vi "refresh table model.vi"(7 "engine configuration":refnum<class "engine configuration.lvclass">, 8 "error in":errorcluster, 9 "avail tags":refnum<vi>, 10 "chan table":refnum<vi>, 11 "TDMS datalogger configuration":refnum<class "TDMS datalogger configuration.lvclass">) -> (0 "error out":errorcluster, 3 "TDMS datalogger configuration out":refnum<class "TDMS datalogger configuration.lvclass">, 5 "engine configuration out":refnum<class "engine configuration.lvclass">)   [LabVIEW 2013, in "TDMS datalogger editor node.lvclass"]
uses:
  TDMS datalogger editor node.lvclass
  <vilib>/NI/TBM Modules/TDMS Datalogger/module/configuration/TDMS datalogger configuration.lvclass
  <vilib>/NI/Module Execution Interface/Engine Configuration/engine configuration.lvclass
  <vilib>/NI/Tag Bus Module Framework/root configuration/TBM configuration.lvclass/TBM configuration.ctl
  <vilib>/NI/TBM Modules/TDMS Datalogger/module/configuration/TDMS datalogger configuration.lvclass/TDMS datalogger configuration.ctl
  <vilib>/NI/Tag Bus/tag/tag descriptor.lvclass/tag descriptor.ctl
  <vilib>/NI/Module Execution Interface/Engine Configuration/engine configuration.lvclass/engine configuration.ctl
  <vilib>/NI/Tag Bus/tag/read tag name.vi
  <vilib>/NI/Tag Bus/tag/read data type.vi
  <vilib>/NI/Tag Bus Module Framework/root configuration/Read instance name.vi
  <vilib>/NI/TBM Modules/TDMS Datalogger/module/configuration/Read channels.vi
  <vilib>/NI/Tag Bus Module Framework/root configuration/create GUID.vi
  <vilib>/NI/Tag Bus Module Framework/channel/TBM channel.lvclass
  <vilib>/NI/Tag Bus/tag/tag descriptor.lvclass
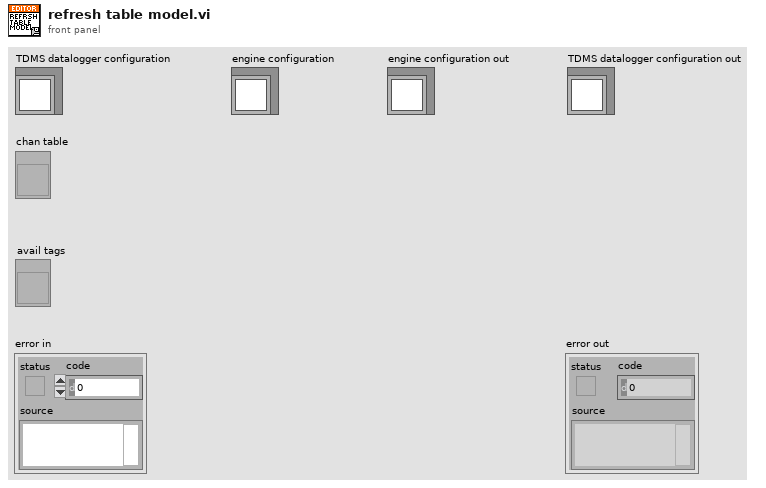
[diagram p1: front panel]
types:
  T1 = typedef "tag bus.lvlib/tag descriptor.lvclass/Data Type.ctl" = enum16{"Double", "Single", "I64", "I32", "I16", "I8", "U64", "U32", "U16", "U8", "Boolean", "String", "Array of Double", "Array of Single", "Array of I64", "Array of I32", "Array of I16", "Array of I8", "Array of U64", "Array of U32", "Array of U16", "Array of U8", "Array of Boolean", "Array of String"}
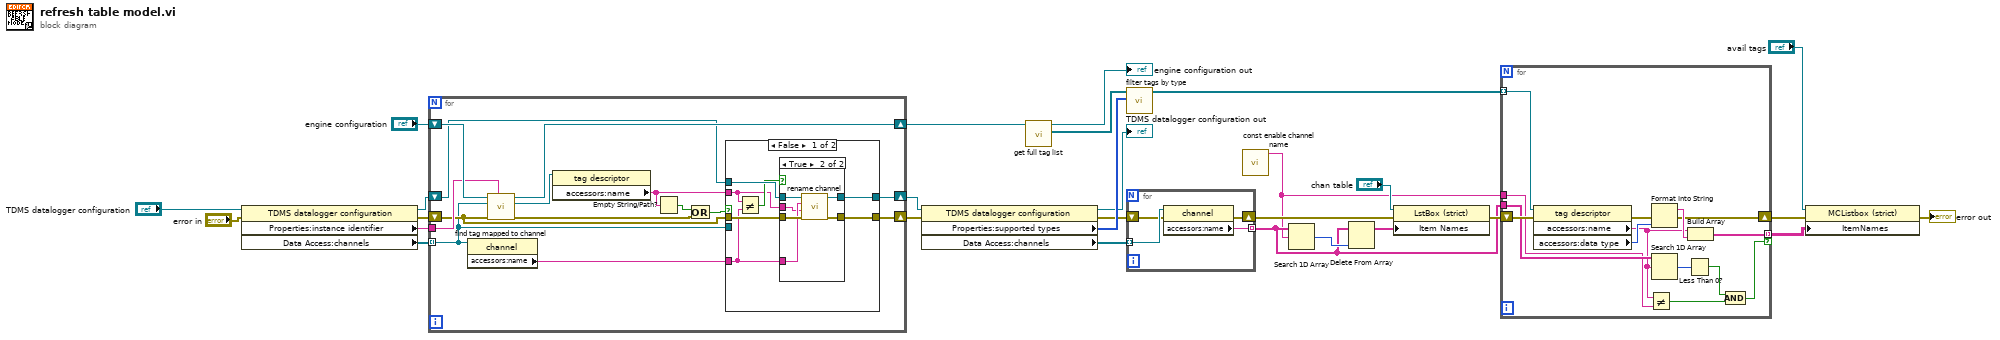
[diagram p0: block diagram]
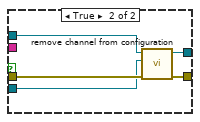
[diagram p3: hidden frame]
diagram:
  n1 = property class="TDMS datalogger configuration"(reference="TDMS datalogger configuration", error in="error in") -> (reference out=w23:refnum<class "TDMS datalogger configuration.lvclass">, error out=w25:errorcluster, "Properties:instance identifier"=w19:string, "Data Access:channels"=w26:refnum<class "TBM channel.lvclass">[])
  n2 = for {
    tunnel: w26 -> [w32] mode=indexing
    shift-right: [w40] -> w5
    shift-left: "engine configuration" -> [w42]
    shift-right: [w37] -> w22
    shift-left: w23 -> [w35]
    tunnel: w19 -> [w41]
    shift-right: [w36] -> w21
    shift-left: w25 -> [w33]
    n3 = property class="channel"(reference=w32) -> ("accessors:name"=w30:string)  [unwired: 1 in, 2 out]
    n4 = call <vilib>:"find tag mapped to channel.vi"("owner"=w41, "error in"=w33, "channel"=w32, "engine configuration in"=w42) -> ("error out"=w31:errorcluster, "tag"=w39:refnum<class "tag descriptor.lvclass">, "engine configuration out"=w40:refnum<class "engine configuration.lvclass">)  [unwired: 5 in]
    n5 = property class="tag descriptor"(reference=w39) -> ("accessors:name"=w29:string)  [unwired: 1 in, 2 out]
    n6 = Empty String/Path?(string/path=w29) -> (empty?=w38:bool)
    n7 = Or(x=w38, y=w31) -> (x .or. y?=w34:bool)
    n8 = case shown="False" w34 {
      tunnel: [w46 w62] -> w37
      tunnel: [w49 w61] -> w36
      tunnel: w33 -> [w48 w60]
      tunnel: w35 -> [w47 w59]
      tunnel: w32 -> [_ w58]
      tunnel: w30 -> [w44 _]
      tunnel: w29 -> [w43 _]
      frame False {
        n9 = Not Equal?(x=w43, y=w44) -> (x != y?=w45:bool)
        n10 = case shown="True" w45 {
          tunnel: [w51 w55] -> w49
          tunnel: w48 -> [w51 w56]
          tunnel: w47 -> [w50 w57]
          tunnel: [w50 w54] -> w46
          tunnel: w44 -> [_ w53]
          tunnel: w43 -> [_ w52]
          frame False {
          }
          frame True {
            n11 = call <vilib>:"rename channel.vi"("error in"=w56, "new name"=w52, "old name"=w53, "TDMS datalogger configuration in"=w57) -> ("error out"=w55:errorcluster, "TDMS datalogger configuration out"=w54:refnum<class "TDMS datalogger configuration.lvclass">)  [unwired: 6 in]
          }
        }
      }
      frame True {
        n12 = call <vilib>:"remove channel from configuration.vi"("error in"=w60, "TBM channel in"=w58, "TDMS datalogger configuration in"=w59) -> ("error out"=w61:errorcluster, "TDMS datalogger configuration out"=w62:refnum<class "TDMS datalogger configuration.lvclass">)  [unwired: 7 in]
      }
    }
  }
  n13 = property class="TDMS datalogger configuration"(reference=w22, error in=w21) -> (reference out=→"TDMS datalogger configuration out":refnum<class "TDMS datalogger configuration.lvclass">, error out=w17:errorcluster, "Properties:supported types"=w20:T1[], "Data Access:channels"=w18:refnum<class "TBM channel.lvclass">[])
  n14 = call <vilib>:"get full tag list.vi"("engine configuration in"=w5) -> ("tag list"=w3:refnum<class "tag descriptor.lvclass">[], "engine configuration out"=→"engine configuration out":refnum<class "engine configuration.lvclass">)  [unwired: 9 in]
  n15 = call <vilib>:"filter tags by type.vi"("allowable types"=w20, "tags in"=w3) -> ("filtered tags"=w14:refnum<class "tag descriptor.lvclass">[])  [unwired: 9 in]
  n16 = for {
    tunnel: w18 -> [w66] mode=indexing
    shift-right: [w65] -> w13
    shift-left: w17 -> [w64]
    tunnel: [w63] -> w2 mode=indexing
    n17 = property class="channel"(reference=w66, error in=w64) -> (error out=w65:errorcluster, "accessors:name"=w63:string)  [unwired: 1 out]
  }
  n18 = call <vilib>:"const enable channel name.vi"() -> ("enable channel"=w1:string)  [unwired: 11 in]
  n19 = Search 1D Array(1D array=w2, element=w1) -> (index of element=w16:i32)  [unwired: 1 in]
  n20 = Delete From Array(array=w2, index=w16) -> (array with subset deleted=w15:string[])  [unwired: 1 in, 1 out]
  n21 = property class="LstBox (strict)"(reference="chan table", error in=w13, "Item Names"=w15) -> (error out=w12:errorcluster)  [unwired: 1 out]
  n22 = for {
    tunnel: w14 -> [w78] mode=indexing
    shift-right: [w75] -> w11
    shift-left: w12 -> [w77]
    tunnel: [w74] -> w10 mode=indexing if=w70
    tunnel: w2 -> [w73]
    tunnel: w1 -> [w68]
    n23 = property class="tag descriptor"(reference=w78, error in=w77) -> (error out=w76:errorcluster, "accessors:name"=w69:string, "accessors:data type"=w79:T1)  [unwired: 1 out]
    n24 = Not Equal?(x=w69, y=w68) -> (x != y?=w67:bool)
    n25 = Format Into String(error in=w76, w79) -> (resulting string=w80:string, error out=w75:errorcluster)  [unwired: 2 in]
    n26 = Search 1D Array(1D array=w73, element=w69) -> (index of element=w72:i32)  [unwired: 1 in]
    n27 = Less Than 0?(x=w72) -> (x < 0?=w71:bool)
    n28 = Build Array(w69, w80) -> (w74:string[])
    n29 = Compound Arithmetic op=AND(w71, w67) -> (w70:bool)
  }
  n30 = property class="MCListbox (strict)"(reference="avail tags", error in=w11, "ItemNames"=w10) -> (error out=→"error out":errorcluster)  [unwired: 1 out]
